vi "ReadCamCal.vi"   [LabVIEW 2016]
uses:
  <vilib>/Utility/config.llb/Read Key (Double).vi
  <vilib>/Rock Robotics/Network Tables/NT Write Number.vi
  <vilib>/Utility/config.llb/NI_LVConfig.lvlib
types:
  T1 = typedef "NI_LVConfig.lvlib/Config Data RefNum.ctl" = refnum<k1>
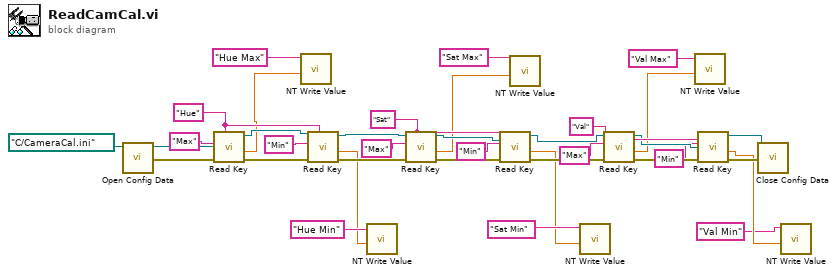
[diagram p0: block diagram]
diagram:
  w23 = "Val" ("section")
  w24 = "Sat" ("section")
  w36 = "Hue" ("section")
  n1 = call <vilib>:"Open Config Data.vi"("configuration file path"=path "C:/CameraCal.ini") -> ("error out"=w31:errorcluster, "refnum"=w30:T1)  [unwired: 8 in, 1 out]
  n2 = call-poly <vilib>:"Read Key.vi"("section"=w36, "error in (no error)"=w31, "key"="Max", "refnum"=w30) -> ("error out"=w35:errorcluster, "value"=w11:dbl, "refnum out"=w34:T1)  [unwired: 4 in, 1 out]
  n3 = call-poly <vilib>:"NT Write Value.vi"("Numeric"=w11, "Name"="Hue Max" ("section")) -> ()  [unwired: 9 in, 1 out]
  n4 = call-poly <vilib>:"Read Key.vi"("section"=w36, "error in (no error)"=w35, "key"="Min", "refnum"=w34) -> ("error out"=w17:errorcluster, "value"=w9:dbl, "refnum out"=w18:T1)  [unwired: 4 in, 1 out]
  n5 = call-poly <vilib>:"NT Write Value.vi"("Numeric"=w9, "Name"="Hue Min" ("section")) -> ()  [unwired: 9 in, 1 out]
  n6 = call-poly <vilib>:"Read Key.vi"("section"=w24, "error in (no error)"=w17, "key"="Max", "refnum"=w18) -> ("error out"=w25:errorcluster, "value"=w8:dbl, "refnum out"=w26:T1)  [unwired: 4 in, 1 out]
  n7 = call-poly <vilib>:"Read Key.vi"("section"=w24, "error in (no error)"=w25, "key"="Min", "refnum"=w26) -> ("error out"=w15:errorcluster, "value"=w5:dbl, "refnum out"=w16:T1)  [unwired: 4 in, 1 out]
  n8 = call-poly <vilib>:"NT Write Value.vi"("Numeric"=w8, "Name"="Sat Max" ("section")) -> ()  [unwired: 9 in, 1 out]
  n9 = call-poly <vilib>:"NT Write Value.vi"("Numeric"=w5, "Name"="Sat Min" ("section")) -> ()  [unwired: 9 in, 1 out]
  n10 = call-poly <vilib>:"Read Key.vi"("section"=w23, "error in (no error)"=w15, "key"="Max", "refnum"=w16) -> ("error out"=w22:errorcluster, "value"=w4:dbl, "refnum out"=w21:T1)  [unwired: 4 in, 1 out]
  n11 = call-poly <vilib>:"NT Write Value.vi"("Numeric"=w4, "Name"="Val Max" ("section")) -> ()  [unwired: 9 in, 1 out]
  n12 = call-poly <vilib>:"Read Key.vi"("section"=w23, "error in (no error)"=w22, "key"="Min", "refnum"=w21) -> ("error out"=w14:errorcluster, "value"=w2:dbl, "refnum out"=w13:T1)  [unwired: 4 in, 1 out]
  n13 = call <vilib>:"Close Config Data.vi"("error in (no error)"=w14, "refnum"=w13) -> ()  [unwired: 8 in, 2 out]
  n14 = call-poly <vilib>:"NT Write Value.vi"("Numeric"=w2, "Name"="Val Min" ("section")) -> ()  [unwired: 9 in, 1 out]
